vi "Finish.vi"   [LabVIEW 2019]
doc: "This VI is called just before exiting. It is expected to close I/O refnum, save collected data, etc."
uses:
  RobotGlobal.vi
  Classes/Robot/Robot.lvclass
  Classes/Pnematics control/Pneumatics.lvclass
  Classes/DriveOld/Drive.lvclass
  Classes/Vision/Vision.lvclass
  Classes/Cargo/Cargo.lvclass
  Classes/Elevator/Elevator.lvclass
  Classes/Hatch/Hatch.lvclass
  Classes/Joysticks/Joysticks.lvclass
types:
  T1 = typedef "RobotObjects.ctl" = cluster{"Drive.lvclass":refnum<class "Tank Drive.lvclass">, "Pneumatics.lvclass":refnum<class "Pneumatics.lvclass">, "Vision.lvclass":refnum<class "Vision.lvclass">, "Joysticks.lvclass":refnum<class "Joysticks.lvclass">, "Elevator.lvclass":refnum<class "Elevator.lvclass">, "Hatch.lvclass":refnum<class "Hatch.lvclass">, "Cargo.lvclass":refnum<class "Cargo.lvclass">, "DriveOld.lvclass":refnum<class "Drive.lvclass">, "Robot.lvclass":refnum<class "Robot.lvclass">}
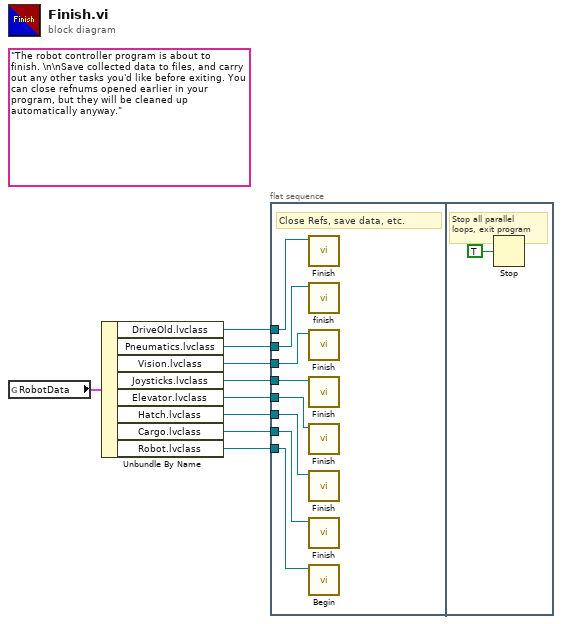
[diagram p0: block diagram]
diagram:
  (unwired) "The robot controller program is about to finish. \n\nSave collected data to files, and carry out any other tasks you'd like before exiting. You can close refnums opened earlier in your program, but they will be cleaned up automatically anyway."
  n1 = global read "RobotGlobal.vi" "RobotData"() -> (w9:T1)
  n2 = Unbundle By Name(w9) -> ("DriveOld.lvclass"=w7:refnum<class "Drive.lvclass">, "Pneumatics.lvclass"=w8:refnum<class "Pneumatics.lvclass">, "Vision.lvclass"=w6:refnum<class "Vision.lvclass">, "Joysticks.lvclass"=w4:refnum<class "Joysticks.lvclass">, "Elevator.lvclass"=w2:refnum<class "Elevator.lvclass">, "Hatch.lvclass"=w3:refnum<class "Hatch.lvclass">, "Cargo.lvclass"=w5:refnum<class "Cargo.lvclass">, "Robot.lvclass"=w1:refnum<class "Robot.lvclass">)
  n3 = flat-sequence {
    tunnel: w8 -> [w17]
    tunnel: w7 -> [w16]
    tunnel: w6 -> [w15]
    tunnel: w5 -> [w14]
    tunnel: w4 -> [w13]
    tunnel: w3 -> [w12]
    tunnel: w2 -> [w11]
    tunnel: w1 -> [w10]
    frame #0 {
      # "Close Refs, save data, etc."
      n4 = call-dynamic "Finish.vi"("Drive in"=w16) -> ()  [unwired: 9 in, 2 out]
      n5 = call-dynamic "finish.vi"("Pneumatics in"=w17) -> ()  [unwired: 9 in, 2 out]
      n6 = call-dynamic "Finish.vi"("Vision in"=w15) -> ()  [unwired: 9 in, 2 out]
      n7 = call-dynamic "Finish.vi"("Joysticks in"=w13) -> ()  [unwired: 9 in, 2 out]
      n8 = call-dynamic "Finish.vi"("Elevator in"=w11) -> ()  [unwired: 9 in, 2 out]
      n9 = call-dynamic "Finish.vi"("Hatch in"=w12) -> ()  [unwired: 9 in, 2 out]
      n10 = call-dynamic "Finish.vi"("Cargo in"=w14) -> ()  [unwired: 9 in, 2 out]
      n11 = call-dynamic "Begin.vi"("Robot in"=w10) -> ()  [unwired: 9 in, 2 out]
    }
    frame #1 {
      # "Stop all parallel\nloops, exit program"
      n12 = Stop(stop? (T)=TRUE ("Quit")) -> ()
    }
  }
